vi "Seek Audio.vi"(7 "Audio CFG in":T1 {"task ID" format="%.0x"}, 8 "error in (no error)":errorcluster, 11 "Seek Position %":dbl) -> (0 "error out":errorcluster, 4 "Now Playing (%)":dbl, 5 "Audio CFG out":T1 {"task ID" format="%.0x"}, 6 "Now Playing (Time)":string)   [LabVIEW 2020]
uses:
  typedefs/Audio CFG.ctl
  <vilib>/Dataflow_G/G-Audio/Controls/Audio File Info.ctl
  <vilib>/sound2/lvsound2.llb/Sound Output Task ID.ctl
  Result To Error - Copy.vi
  <vilib>/Utility/error.llb/Error Cluster From Error Code.vi
  <vilib>/Dataflow_G/G-Audio/G-Audio.lvlib
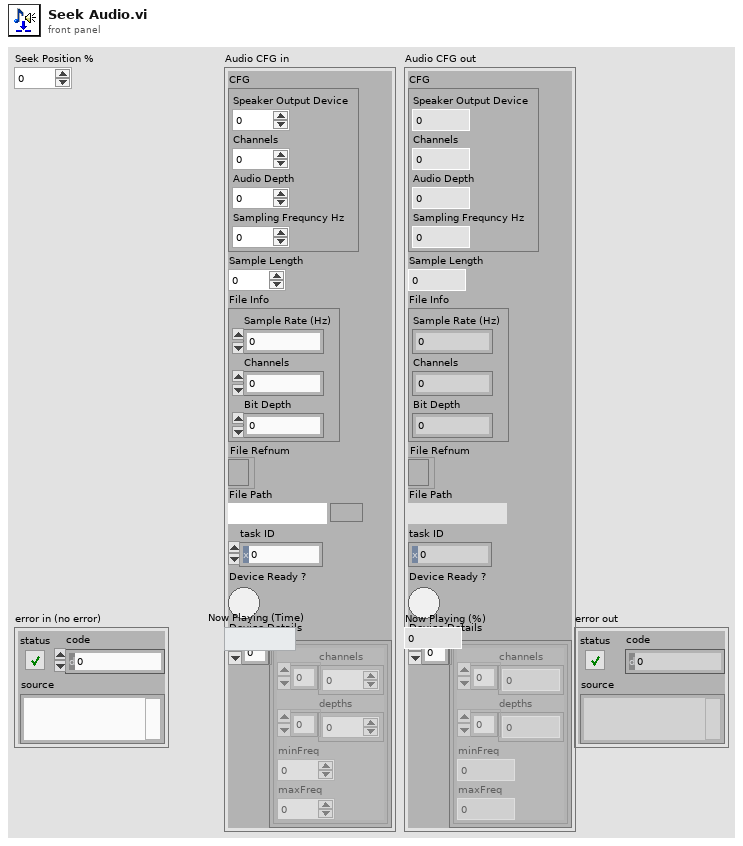
[diagram p1: front panel]
types:
  T1 = typedef "Audio CFG.ctl" = cluster{"CFG":cluster{"Speaker Output Device":u32, "Channels":i32, "Audio Depth":i32, "Sampling Frequncy Hz":dbl}, "Sample Length":u64, "File Info":T2, "File Refnum":refnum<file>, "File Path":path, "Task ID":T3, "Device Ready ?":bool, "Device Details":cluster{"channels":i32[], "depths":i32[], "minFreq":dbl, "maxFreq":dbl}[]}
  T2 = typedef "G-Audio.lvlib/Audio File Info.ctl" = cluster{"Sample Rate (Hz)":u32, "Channels":u32, "Bit Depth":u32}
  T3 = typedef "Sound Output Task ID.ctl" = u32
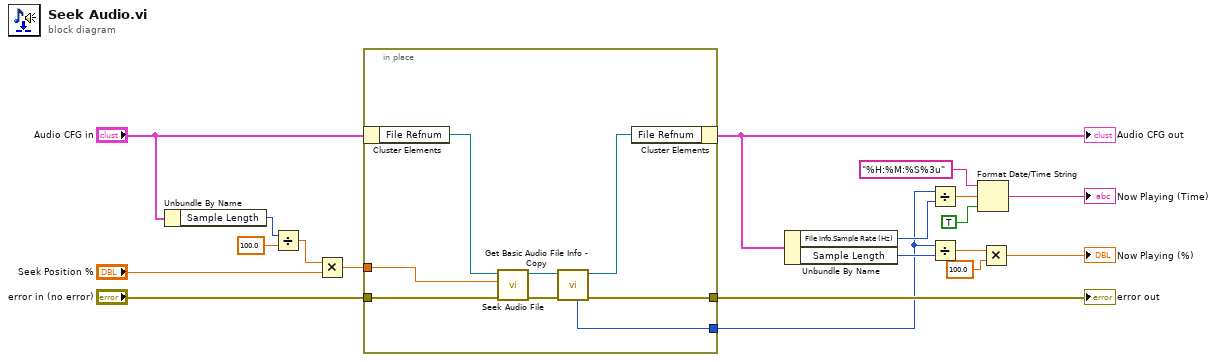
[diagram p0: block diagram]
diagram:
  n1 = Unbundle By Name("Audio CFG in") -> ("Sample Length"=w13:u64)
  n2 = Divide(x=w13, y=100.0) -> (x/y=w15:dbl)
  n3 = Multiply(x=w15, y="Seek Position %") -> (x*y=w18:dbl)
  n4 = in-place {
    in-place-border: "error in (no error)" -> [w27]
    in-place-border: [w23] -> w17
    in-place-border: w18 -> [w25]
    in-place-border: [w20] -> w2
    n5 = in-place-cluster #1("Audio CFG in") -> ("File Refnum"=w24:refnum<file>)
    n6 = call <vilib>:"Seek Audio File.vi"("error in (no error)"=w27, "Seek Position"=w25, "Audio File Refnum In"=w24) -> ("error out"=w26:errorcluster, "Audio File Refnum Out"=w22:refnum<file>)  [unwired: 7 in]
    n7 = call "Get Basic Audio File Info - Copy.vi"("error in (no error)"=w26, "Audio File Refnum In"=w22) -> ("error out"=w23:errorcluster, "Audio File Refnum Out"=w21:refnum<file>, "read_offset"=w20:u64)  [unwired: 5 in, 2 out]
    n8 = in-place-cluster #1("File Refnum"=w21) -> (w3:T1)
  }
  "Audio CFG out" <- w3
  "error out" <- w17
  n9 = Unbundle By Name(w3) -> ("File Info.Sample Rate (Hz)"=w8:u32, "Sample Length"=w7:u64)
  n10 = Divide(x=w2, y=w8) -> (x/y=w10:dbl)
  n11 = Divide(x=w2, y=w7) -> (x/y=w6:dbl)
  n12 = Format Date/Time String(time format string (%c)="%H:%M:%S%3u", seconds (now)=w10, UTC format=TRUE) -> (date/time string=→"Now Playing (Time)":string)
  n13 = Multiply(x=w6, y=100.0) -> (x*y=→"Now Playing (%)":dbl)
